vi "Fix Timestamp.vi"(8 "error in (no error)":errorcluster, 10 "Timestamp in":dbl, 11 "GroupAbstract in":refnum<class "GroupAbstract.lvclass">) -> (0 "error out":errorcluster, 2 "Timestamp":dbl, 3 "GroupAbstract out":refnum<class "GroupAbstract.lvclass">)   [LabVIEW 2020, in "Vecto.lvlib" / "GroupAbstract.lvclass"]
uses:
  GroupAbstract.lvclass
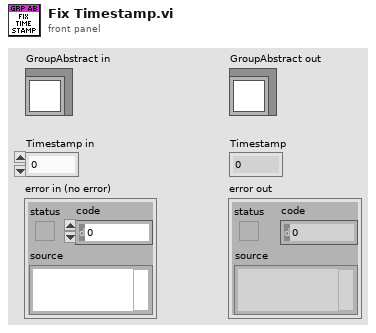
[diagram p1: front panel]
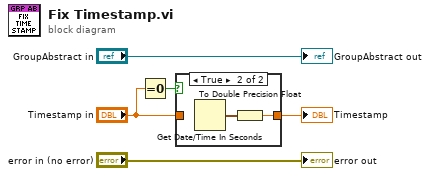
[diagram p0: block diagram]
diagram:
  n1 = Equal To 0?(x="Timestamp in") -> (x = 0?=w3:bool)
  n2 = case shown="True" w3 {
    tunnel: "Timestamp in" -> [w6 _]
    tunnel: [w6 w7] -> w1
    frame False {
    }
    frame True {
      n3 = Get Date/Time In Seconds() -> (seconds since 1Jan1904=w8:timestamp)
      n4 = To Double Precision Float(number=w8) -> (double precision float=w7:dbl)
    }
  }
  "Timestamp" <- w1
  "error out" <- "error in (no error)"
  "GroupAbstract out" <- "GroupAbstract in"
